vi "create_data_folders.vi"(9 "Date array":string[](array[string]), 10 "Experiment Indicator":string, 11 "username":string) -> (3 "Data Output Folder":path)   [LabVIEW 2016]
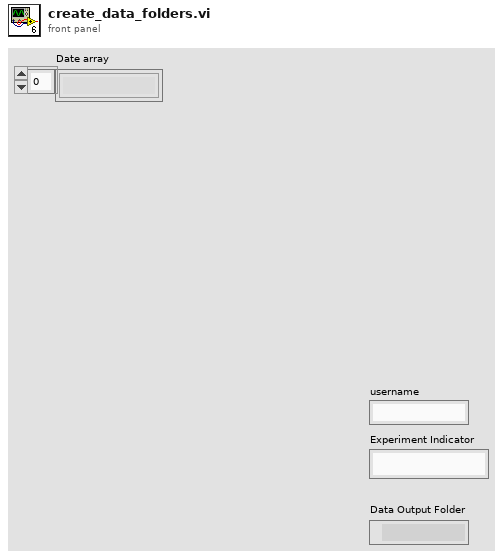
[diagram p1: front panel]
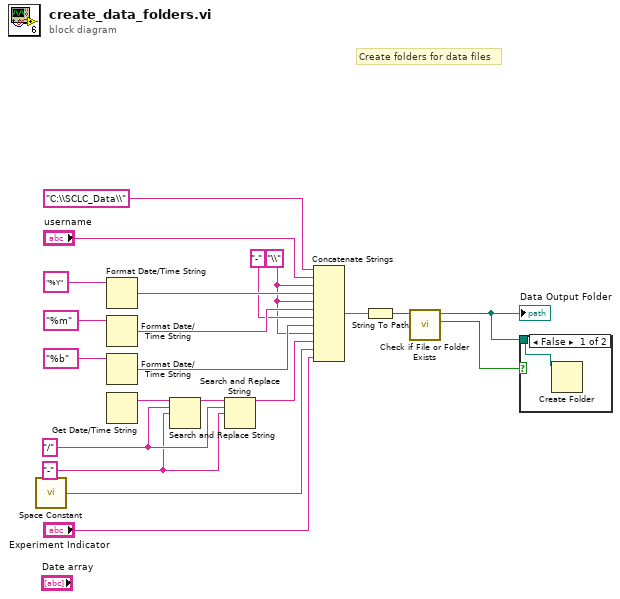
[diagram p0: block diagram]
diagram:
  w9 = "-"
  w10 = "/"
  w4 = "\\"
  # "Create folders for data files"
  n1 = call <vilib>:"Space Constant.vi"() -> ("String"=w2:string)
  n2 = Format Date/Time String(time format string (%c)="%Y") -> (date/time string=w8:string)  [unwired: 2 in]
  n3 = Format Date/Time String(time format string (%c)="%m") -> (date/time string=w7:string)  [unwired: 2 in]
  n4 = Format Date/Time String(time format string (%c)="%b") -> (date/time string=w5:string)  [unwired: 2 in]
  n5 = Get Date/Time String() -> (date string=w12:string)  [unwired: 3 in, 1 out]
  n6 = Search and Replace String(input string=w12, search string=w10, replace string=w9) -> (result string=w11:string)  [unwired: 5 in, 3 out]
  n7 = Search and Replace String(input string=w11, search string=w10, replace string=w9) -> (result string=w3:string)  [unwired: 5 in, 3 out]
  n8 = Concatenate Strings("C:\\SCLC_Data\\", "username", w4, w8, w4, w7, "-", w5, w4, w3, w2, "Experiment Indicator") -> (w17:string)
  n9 = String To Path(string=w17) -> (path=w20:path)
  n10 = call <vilib>:"Check if File or Folder Exists.vi"("path"=w20) -> ("file or folder exists?"=w21:bool, "dup path"=w16:path)  [unwired: 8 in, 1 out]
  "Data Output Folder" <- w16
  n11 = case shown="False" w21 {
    tunnel: w16 -> [w22 _]
    frame False {
      n12 = Create Folder(path (use dialog)=w22) -> ()  [unwired: 2 in, 3 out]
    }
    frame True {
    }
  }
